vi "Refresh Role.vi"(8 "error in (no error)":errorcluster, 11 "PluginGUI in":refnum<class "PluginGUI.lvclass">) -> (0 "error out":errorcluster, 3 "PluginGUI out":refnum<class "PluginGUI.lvclass">)   [LabVIEW 2020, in "VolatusGUI.lvlib" / "PluginGUI.lvclass"]
uses:
  PluginGUI.lvclass
  PluginGUI.lvclass/PluginGUI.ctl
  Volatus/Roles API/Roles API.lvclass/Roles API.ctl
  GUI Element/GUI Element.lvclass/GUI Element.ctl
  GUI Element/GUI Element.lvclass
  Volatus/Roles API/Roles API.lvclass
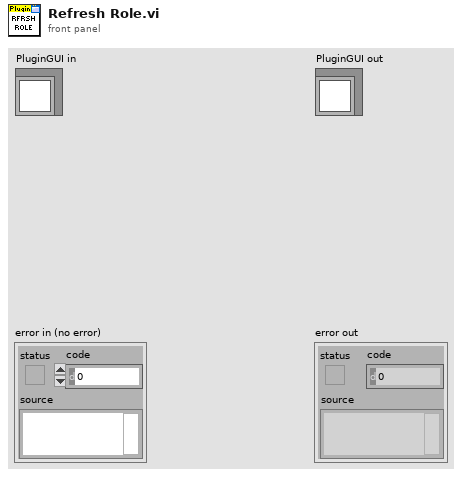
[diagram p1: front panel]
types:
  T1 = enum8{"Enabled", "Disabled", "Disabled and Grayed Out"}
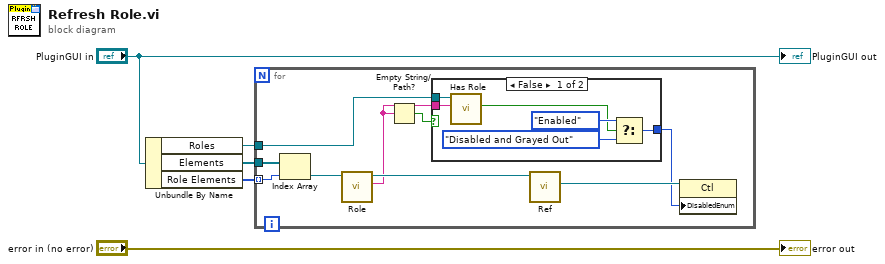
[diagram p0: block diagram]
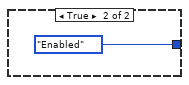
[diagram p2: hidden frame]
diagram:
  n1 = Unbundle By Name("PluginGUI in") -> ("Roles"=w2:refnum<class "Roles API.lvclass">, "Elements"=w3:refnum<class "GUI Element.lvclass">[], "Role Elements"=w1:i32[])
  n2 = for {
    tunnel: w3 -> [w8]
    tunnel: w2 -> [w13]
    tunnel: w1 -> [w7] mode=indexing
    n3 = Index Array(array=w8, index=w7) -> (element=w6:refnum<class "GUI Element.lvclass">)
    n4 = call "Role.vi"("GUI Element in"=w6) -> ("Role"=w11:string, "GUI Element out"=w14:refnum<class "GUI Element.lvclass">)  [unwired: 9 in]
    n5 = Empty String/Path?(string/path=w11) -> (empty?=w10:bool)
    n6 = case shown="False" w10 {
      tunnel: w13 -> [w20 _]
      tunnel: w11 -> [w19 _]
      tunnel: [w15 T1."Enabled" ("Disabled")] -> w9
      frame False {
        n7 = call "Has Role.vi"("Role"=w19, "Roles API in"=w20) -> ("Has Role"=w16:bool)  [unwired: 7 in, 2 out]
        n8 = Select(t=T1."Enabled" ("Disabled"), s=w16, f=T1."Disabled and Grayed Out" ("Disabled")) -> (s? t:f=w15:T1)
      }
      frame True {
      }
    }
    n9 = call "Ref.vi"("GUI Element in"=w14) -> ("Ref"=w12:refnum<vi>)  [unwired: 9 in, 1 out]
    n10 = property class="Ctl"(reference=w12, "DisabledEnum"=w9) -> ()  [unwired: 1 in, 2 out]
  }
  "error out" <- "error in (no error)"
  "PluginGUI out" <- "PluginGUI in"
